vi "config get RunAsService.vi"(5 "Config Keys":T1) -> (2 "RunAsService?":bool)   [LabVIEW 2011]
uses:
  Addons/internet/utils/keyedarr.llb/Keyed Array.ctl
  Addons/internet/utils/strutil.llb/Case Matching.ctl
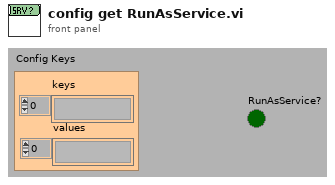
[diagram p1: front panel]
types:
  T1 = typedef "Keyed Array.ctl" = cluster{"keys":string[], "values":string[]}
  T2 = typedef "Case Matching.ctl" = enum16{"a != A", "a == A", "system"}
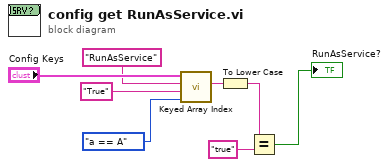
[diagram p0: block diagram]
diagram:
  n1 = call "Keyed Array Index.vi"("case matching (sensitive)"=Case_Matching."a == A", "default value"="True", "key"="RunAsService", "array in"="Config Keys") -> ("value"=w4:string)  [unwired: 3 out]
  n2 = To Lower Case(string=w4) -> (all lower case string=w2:string)
  n3 = Equal?(x=w2, y="true") -> (x = y?=→"RunAsService?":bool)
